vi "Cartesian to Polar.vi"(2 "y":dbl, 3 "x":dbl) -> (0 "magnitude":dbl, 1 "angle":dbl)   [LabVIEW 2014]
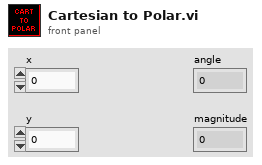
[diagram p1: front panel]
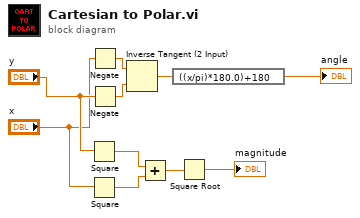
[diagram p0: block diagram]
diagram:
  n1 = Square(x="y") -> (x^2=w6:dbl)
  n2 = Square(x="x") -> (x^2=w5:dbl)
  n3 = Negate(x="x") -> (-x=w8:dbl)
  n4 = Negate(x="y") -> (-x=w7:dbl)
  n5 = Inverse Tangent (2 Input)(1:w7, 2:w8) -> (0:w10:dbl)
  n6 = Add(x=w6, y=w5) -> (x+y=w2:dbl)
  n7 = expression code="((x/pi)*180.0)+180" ("radians to degrees")(w10) -> (→"angle":dbl)
  n8 = Square Root(x=w2) -> (sqrt(x)=→"magnitude":dbl)
